vi "Control Pressure Regulator.vi"(4 "Timeout":i32=30, 6 "y":dbl=0.05 format="%#_13g", 8 "error in":errorcluster, 11 "Desired PSI":dbl) -> (0 "error out":errorcluster, 3 "Reached Setpoint?":bool)   [LabVIEW 2015]
uses:
  <vilib>/DAQmx/write.llb/DAQmx Write (Analog DBL 1Chan 1Samp).vi
  <vilib>/DAQmx/read.llb/DAQmx Read (Analog DBL 1Chan 1Samp).vi
panel:
  out "NI-DAQ Pressure":dbl
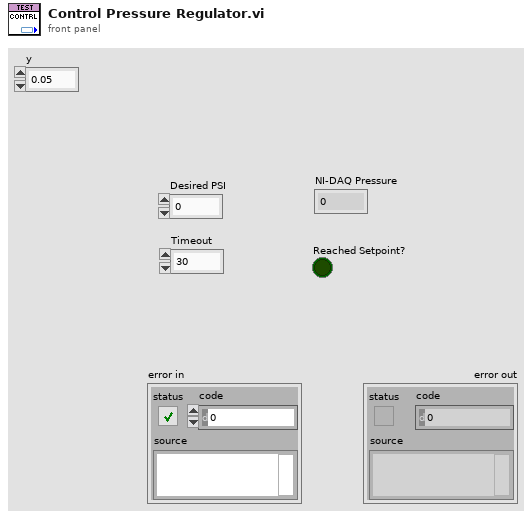
[diagram p1: front panel]
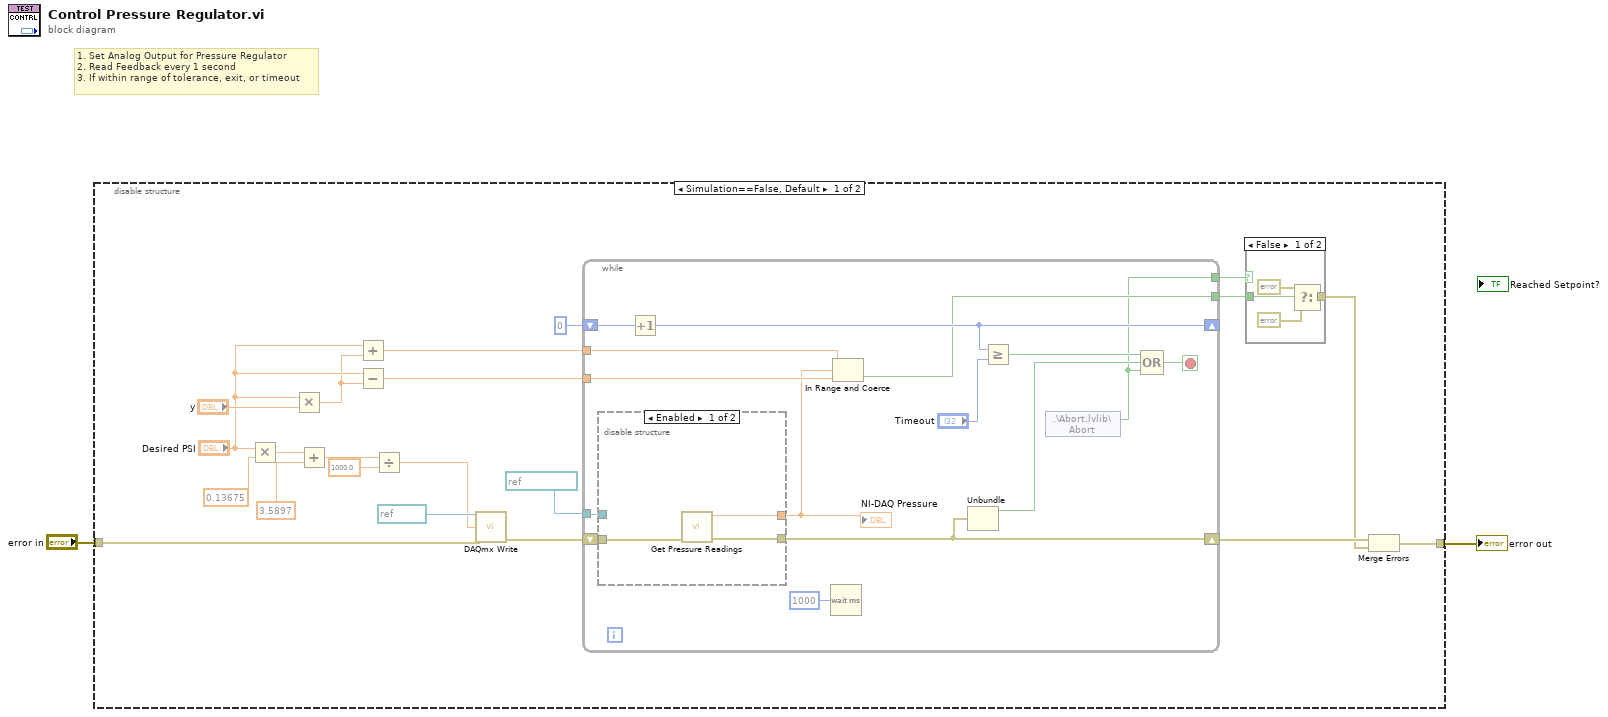
[diagram p0: block diagram]
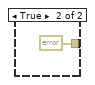
[diagram p2: hidden frame]
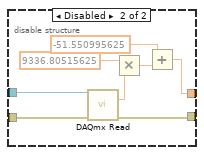
[diagram p3: hidden frame]
diagram:
  # "1. Set Analog Output for Pressure Regulator\n2. Read Feedback every 1 second\n3. If within range of tolerance, exit, or timeout"
  n1 = disable-structure shown="Simulation==False, Default" {
    disable-tunnel: [w9 w55] -> w2
    disable-tunnel: "error in" -> [w3 w55]
    frame condition #0 {
      n2 = Multiply(x="Desired PSI", y=0.13675) -> (x*y=w22:dbl)
      n3 = Multiply(x="Desired PSI", y="y") -> (x*y=w7:dbl)
      n4 = Add(x=w22, y=3.5897) -> (x+y=w19:dbl)
      n5 = Add(x="Desired PSI", y=w7) -> (x+y=w8:dbl)
      n6 = Subtract(x="Desired PSI", y=w7) -> (x-y=w13:dbl)
      n7 = Divide(x=w19, y=1000.0) -> (x/y=w17:dbl)
      n8 = call-poly <vilib>:"DAQmx Write.vi"("task/channels in"=refnum<k21> "REG", "data"=w17, "error in"=w3) -> ("error out"=w15:errorcluster)  [unwired: 10 in, 2 out]
      n9 = while {
        tunnel: refnum<k21> "Pressure" -> [w30]
        shift-right: [w33] -> w5
        shift-left: w15 -> [w34]
        tunnel: w13 -> [w42]
        tunnel: w8 -> [w43]
        shift-right: [w38] -> _
        shift-left: 0 -> [w39]
        tunnel: [w31] -> w10
        tunnel: [w29] -> w6
        stop <- w40 stop-if-true
        n10 = disable-structure shown="Enabled" {
          disable-tunnel: w34 -> [w46 w53]
          disable-tunnel: [w45 w52] -> w33
          disable-tunnel: [w44 w47] -> w32
          disable-tunnel: w30 -> [_ w54]
          frame Enabled {
            n11 = call "Get Pressure Readings.vi"("error in (no error)"=w46) -> ("error out"=w45:errorcluster, "NI-DAQ Pressure"=w44:dbl)  [unwired: 7 in, 2 out]
          }
          frame Disabled {
            n12 = call-poly <vilib>:"DAQmx Read.vi"("task/channels in"=w54, "error in"=w53) -> ("data"=w51:dbl, "error out"=w52:errorcluster)  [unwired: 11 in, 1 out]
            n13 = Multiply(x=9336.80515625 ("y"), y=w51) -> (x*y=w49:dbl)
            n14 = Add(x=-51.550995625, y=w49) -> (x+y=w47:dbl)
          }
        }
        "NI-DAQ Pressure" <- w32
        n15 = Increment(x=w39) -> (x+1=w38:i32)
        n16 = Wait (ms)(milliseconds to wait=u32 1000) -> ()  [unwired: 1 out]
        n17 = In Range and Coerce(upper limit=w43, x=w32, lower limit=w42) -> (In Range?=w31:bool)  [unwired: 1 out]
        n18 = Unbundle(w33) -> ("status"=w41:bool)  [unwired: 2 out]
        n19 = Greater Or Equal?(x=w38, y="Timeout") -> (x >= y?=w35:bool)
        n20 = shared-variable ".\\Abort.lvlib\\Abort"() -> (w29:bool)  [unwired: 1 in, 1 out]
        n21 = Compound Arithmetic op=OR(w35, w41, w29) -> (w40:bool)
      }
      n22 = case shown="False" w6 {
        tunnel: w10 -> [w27 _]
        tunnel: [w26 errorcluster {"status"=FALSE, "code"=0, "source"=""} ("error out")] -> w4
        frame False {
          n23 = Select(t=errorcluster {"status"=FALSE, "code"=0, "source"=""} ("error out"), s=w27, f=errorcluster {"status"=TRUE, "code"=9000, "source"="Timeout Error. Pressure Regulator Failed to Reach Setpoint"} ("error out")) -> (s? t:f=w26:errorcluster)
        }
        frame True {
        }
      }
      n24 = Merge Errors(w5, w4) -> (w9:errorcluster)
    }
    frame condition #1 (active) {
    }
  }
  "error out" <- w2
